vi "roboRIO v1.0 Build MUX Configuration RSL.vi"(11 "RSL Channel List":T4) -> (3 "Channel Reservation List":T1)   [LabVIEW 2021]
uses:
  <vilib>/myRIO/Common/Instrument Driver Framework/roboRIO v1.0/RSL/typedefs/RSL Channels List.ctl
  <vilib>/myRIO/Common/Instrument Driver Framework/roboRIO v1.0/RSL/typedefs/RSL Channels Enum.ctl
  <vilib>/myRIO/Common/Instrument Driver Framework/roboRIO v1.0/Resource Manager/typedefs/roboRIO v1.0 Channel Reservation List.ctl
  <vilib>/myRIO/Common/Instrument Driver Framework/roboRIO v1.0/Resource Manager/typedefs/roboRIO v1.0 Channel Reservation Info.ctl
  <vilib>/myRIO/Common/Instrument Driver Framework/roboRIO v1.0/Resource Manager/typedefs/roboRIO v1.0 Connector List.ctl
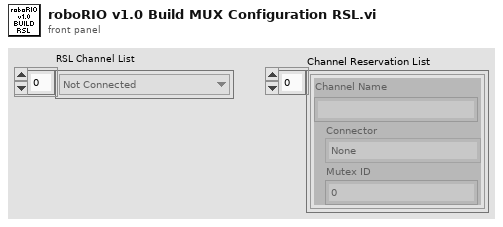
[diagram p1: front panel]
types:
  T1 = typedef "roboRIO v1.0 Channel Reservation List.ctl" = T2[]
  T2 = typedef "roboRIO v1.0 Channel Reservation Info.ctl" = cluster{"Channel Name":string, "Connector":T3, "Mutex ID":i32}
  T3 = typedef "roboRIO v1.0 Connector List.ctl" = enum32{"None", "ConnectorB", "ConnectorI2C", "ConnectorDIO", "ConnectorRSL", "ConnectorRELAY", "ConnectorAI", "ConnectorPWM", "ConnectorSPI"}
  T4 = typedef "RSL Channels List.ctl" = T5[]
  T5 = typedef "RSL Channels Enum.ctl" = enum16{"Not Connected", "RSL/RSL0"}
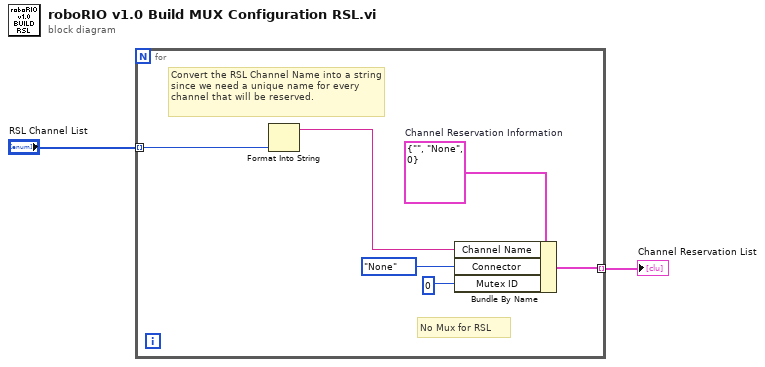
[diagram p0: block diagram]
diagram:
  n1 = for {
    tunnel: "RSL Channel List" -> [w5] mode=indexing
    tunnel: [w7] -> w1 mode=indexing
    w8 = T2 {"Channel Name"="", "Connector"=enum."None", "Mutex ID"=0}  # Channel Reservation Information
    # "Convert the RSL Channel Name into a string since we need a unique name for every channel that will be reserved."
    # "No Mux for RSL"
    n2 = Format Into String(w5) -> (resulting string=w6:string)  [unwired: 3 in, 1 out]
    n3 = Bundle By Name(cluster=w8, "Channel Name"=w6, "Connector"=roboRIO_v1.0_Connector_List."None" ("Connector List"), "Mutex ID"=0) -> (w7:T2)
  }
  "Channel Reservation List" <- w1
